vi "HttpBs.vi"() -> ()   [LabVIEW 2016]
uses:
  <vilib>/httpClient/LabVIEWHTTPClient.lvlib
panel:
  out "Web Request\n Count":i32
  out "Body":string
  out "Header":string
  out "Full URL":string
  in  "stop":bool
  out "Slider Value to write":dbl
  in  "Slider Value":dbl(slide) step=0.1 scale=-10.0..10.0
  in  "String":string
  # "Daniel Smith de Paz"
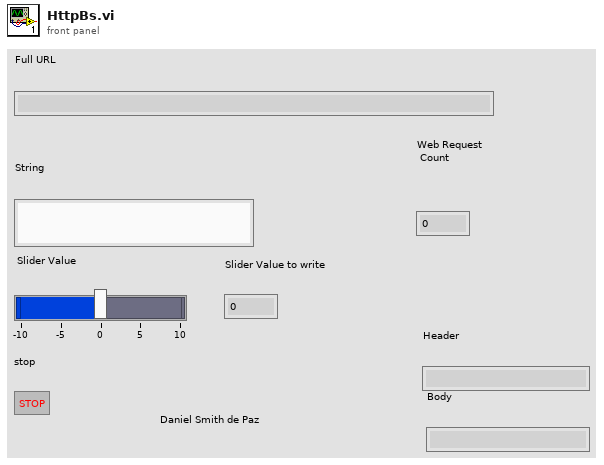
[diagram p1: front panel]
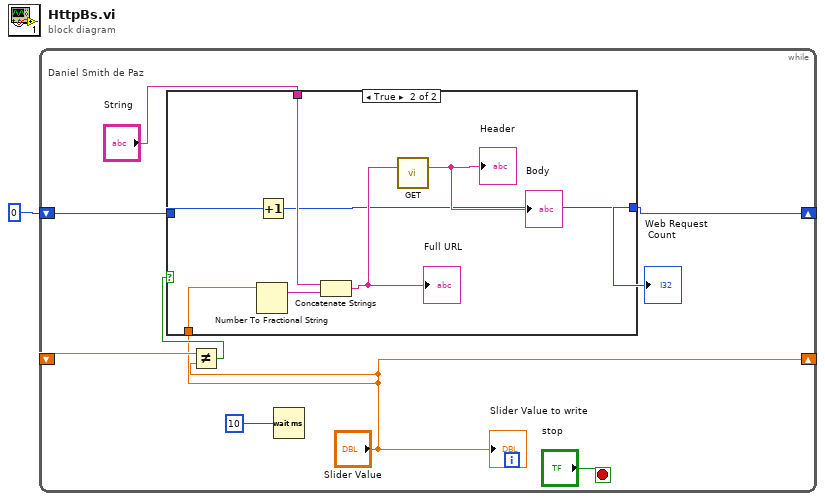
[diagram p0: block diagram]
diagram:
  n1 = while {
    shift-right: ["Slider Value"] -> _
    shift-left: _ -> [w7]
    shift-right: [w3] -> _
    shift-left: 0 -> [w4]
    stop <- "stop" stop-if-true
    # "Daniel Smith de Paz"
    n2 = Not Equal?(x=w7, y="Slider Value") -> (x != y?=w6:bool)
    n3 = case shown="True" w6 {
      tunnel: "String" -> [_ w17]
      tunnel: "Slider Value" -> [_ w15]
      tunnel: [w10 w12] -> w3
      tunnel: w4 -> [w10 w11]
      frame False {
      }
      frame True {
        n4 = Number To Fractional String(number=w15) -> (F-format string=w16:string)  [unwired: 3 in]
        n5 = Increment(x=w11) -> (x+1=w12:i32)
        n6 = Concatenate Strings(w17, w16) -> (w14:string)
        "Full URL" <- w14
        n7 = call <vilib>:"GET.vi"("url"=w14) -> ("headers"=→"Header" →"Body":string)  [unwired: 11 in, 3 out]
      }
    }
    "Web Request\n Count" <- w3
    n8 = Wait (ms)(milliseconds to wait=u32 10) -> ()  [unwired: 1 out]
    "Slider Value to write" <- "Slider Value"
  }
